vi "Write Loop Name.vi"(8 "error in (no error)":errorcluster, 10 "Loop Name":refnum<vi>, 11 "Bioreactor in":refnum<class "Bioreactor.lvclass">) -> (0 "error out":errorcluster, 3 "Bioreactor out":refnum<class "Bioreactor.lvclass">)   [LabVIEW 2013, in "Bioreactor.lvlib" / "Bioreactor.lvclass"]
uses:
  Bioreactor.lvclass
  Bioreactor.lvclass/Bioreactor.ctl
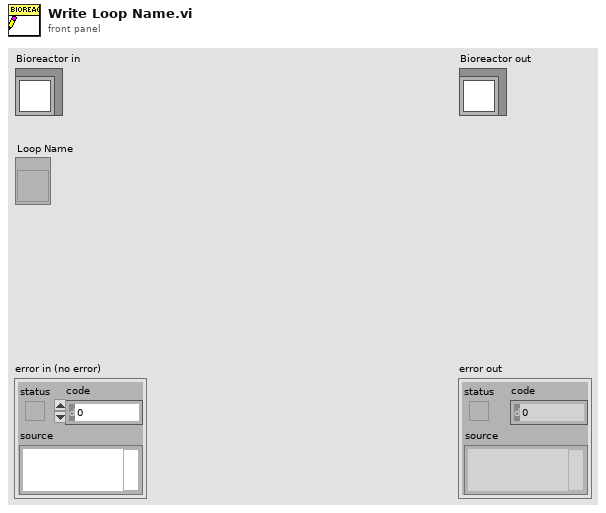
[diagram p1: front panel]
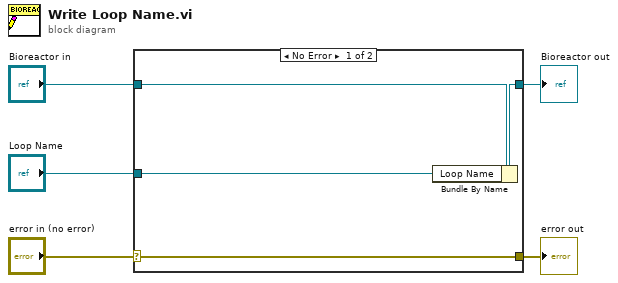
[diagram p0: block diagram]
diagram:
  n1 = case shown="No Error" "error in (no error)" {
    selector: "error in (no error)" -> [w9 w10]
    tunnel: [w9 w10] -> w4
    tunnel: [w7 w11] -> w2
    tunnel: "Bioreactor in" -> [w8 w11]
    tunnel: "Loop Name" -> [w6 _]
    frame No Error {
      n2 = Bundle By Name(cluster=w8, "Loop Name"=w6) -> (w7:refnum<class "Bioreactor.lvclass">)
    }
    frame Error {
    }
  }
  "error out" <- w4
  "Bioreactor out" <- w2
